vi "Rinocloud_metadata_parsing.vi"(8 "error in (no error)":errorcluster, 11 "HTTP body":string) -> (0 "error out":errorcluster, 1 "Notes":string, 2 "Tags":string, 3 "Name":string, 4 "JSON Object":variant, 5 "metadata (JSON)":string)   [LabVIEW 2011, in "Rinocloud Library.lvlib"]
uses:
  Rinocloud Library.lvlib
  i3 JSON/i3-json.lvlib
  i3 JSON/JSON Parsing/Get Object Parameter Files/Get Object Parameter - String.vi
  i3 JSON/JSON Parsing/Get Object Parameter Files/Get Object Parameter - Array.vi
  i3 JSON/JSON Parsing/Get Array Value at Index Files/Get Array Value at Index - String.vi
  i3 JSON/JSON Parsing/Get Object Parameter Files/Get Object Parameter - Object.vi
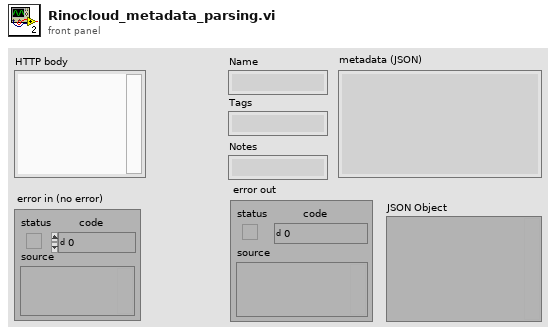
[diagram p1: front panel]
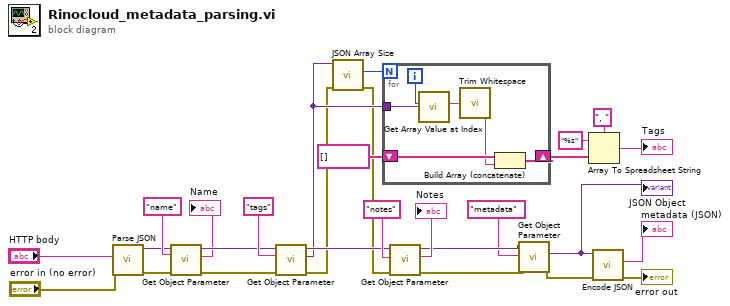
[diagram p0: block diagram]
diagram:
  n1 = call "Parse JSON.vi"("error in (no error)"="error in (no error)", "JSON String"="HTTP body") -> ("error out"=w9:errorcluster, "JSON Tree"=w21:variant)  [unwired: 6 in, 2 out]
  n2 = call-poly "Get Object Parameter.vi"("error in (no error)"=w9, "Parameter Name"="name", "JSON Tree In (JSON Object)"=w21) -> ("error out"=w8:errorcluster, "String Value"=→"Name":string, "JSON Tree Out Passthrough"=w26:variant)  [unwired: 5 in, 1 out]
  n3 = call-poly "Get Object Parameter.vi"("error in (no error)"=w8, "Parameter Name"="tags", "JSON Tree In (JSON Object)"=w26) -> ("error out"=w5:errorcluster, "JSON Array"=w19:variant, "JSON Tree Out Passthrough"=w24:variant)  [unwired: 5 in, 1 out]
  n4 = call "JSON Array Size.vi"("error in (no error)"=w5, "JSON Tree In (JSON Array)"=w19) -> ("error out"=w4:errorcluster, "Array Size"=w20:i32)  [unwired: 7 in, 1 out]
  n5 = for {
    N: w20 -> [_]
    tunnel: w19 -> [w34]
    shift-right: [w32] -> w15
    shift-left: string[] [] ("Tags 2") -> [w33]
    i -> [w31]
    n6 = call-poly "Get Array Value at Index.vi"("Index"=w31, "JSON Tree In (JSON Array)"=w34) -> ("String Value"=w30:string)  [unwired: 6 in, 3 out]
    n7 = call <vilib>:"Trim Whitespace.vi"("string"=w30) -> ("trimmed string"=w29:string)  [unwired: 1 in]
    n8 = Build Array (concatenate)(w33, w29) -> (w32:string[])
  }
  n9 = call-poly "Get Object Parameter.vi"("error in (no error)"=w4, "Parameter Name"="notes", "JSON Tree In (JSON Object)"=w24) -> ("error out"=w7:errorcluster, "String Value"=→"Notes":string, "JSON Tree Out Passthrough"=w13:variant)  [unwired: 5 in, 1 out]
  n10 = call-poly "Get Object Parameter.vi"("error in (no error)"=w7, "Parameter Name"="metadata", "JSON Tree In (JSON Object)"=w13) -> ("error out"=w6:errorcluster, "JSON Object"=w11:variant)  [unwired: 5 in, 2 out]
  "JSON Object" <- w11
  n11 = Array To Spreadsheet String(delimiter (Tab)=", ", array=w15, 3:"%s" ("format string")) -> (spreadsheet string=→"Tags":string)
  n12 = call "Encode JSON.vi"("error in (no error)"=w6, "JSON Tree"=w11) -> ("error out"=→"error out":errorcluster, "String"=→"metadata (JSON)":string)  [unwired: 4 in]
